vi "Calc Distance.vi"(9 "Height":dbl, 10 "Width":dbl, 11 "Focal Length":dbl) -> (2 "Angle":dbl=1.211552449916613, 3 "Distance":dbl=100.14913892002585)   [LabVIEW 2015]
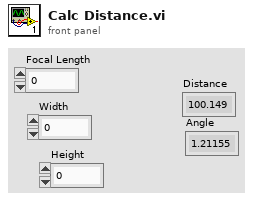
[diagram p1: front panel]
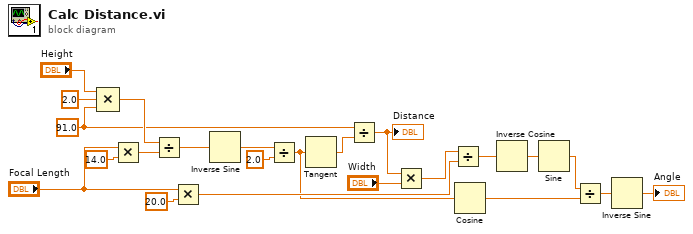
[diagram p0: block diagram]
diagram:
  w16 = 91.0 ("value")
  n1 = Compound Arithmetic op=MULTIPLY("Height", 2.0 ("value"), w16) -> (w20:dbl)
  n2 = Multiply(x="Focal Length", y=14.0) -> (x*y=w19:dbl)
  n3 = Divide(x=w20, y=w19) -> (x/y=w4:dbl)
  n4 = Multiply(x="Focal Length", y=20.0) -> (x*y=w12:dbl)
  n5 = Inverse Sine(1:w4) -> (0:w23:dbl)
  n6 = Divide(x=w23, y=2.0) -> (x/y=w5:dbl)
  n7 = Tangent(1:w5) -> (0:w18:dbl)
  n8 = Divide(x=w16, y=w18) -> (x/y=w14:dbl)
  "Distance" <- w14
  n9 = Multiply(x=w14, y="Width") -> (x*y=w13:dbl)
  n10 = Divide(x=w13, y=w12) -> (x/y=w10:dbl)
  n11 = Cosine(x=w5) -> (cos(x)=w7:dbl)
  n12 = Inverse Cosine(1:w10) -> (0:w9:dbl)
  n13 = Sine(x=w9) -> (sin(x)=w8:dbl)
  n14 = Divide(x=w8, y=w7) -> (x/y=w6:dbl)
  n15 = Inverse Sine(1:w6) -> (0:→"Angle":dbl)
